vi "WRITE CAN DATA DBL.vi"(7 "Enum":T1=enum."GET", 8 "error in (no error)":errorcluster, 11 "CAN DATA IN":dbl[](array[numeric])) -> (0 "error out":errorcluster, 3 "CAN DATA OUT":dbl[](array[numeric]))   [LabVIEW 2018]
uses:
  Controls/READ CAN DATA.ctl
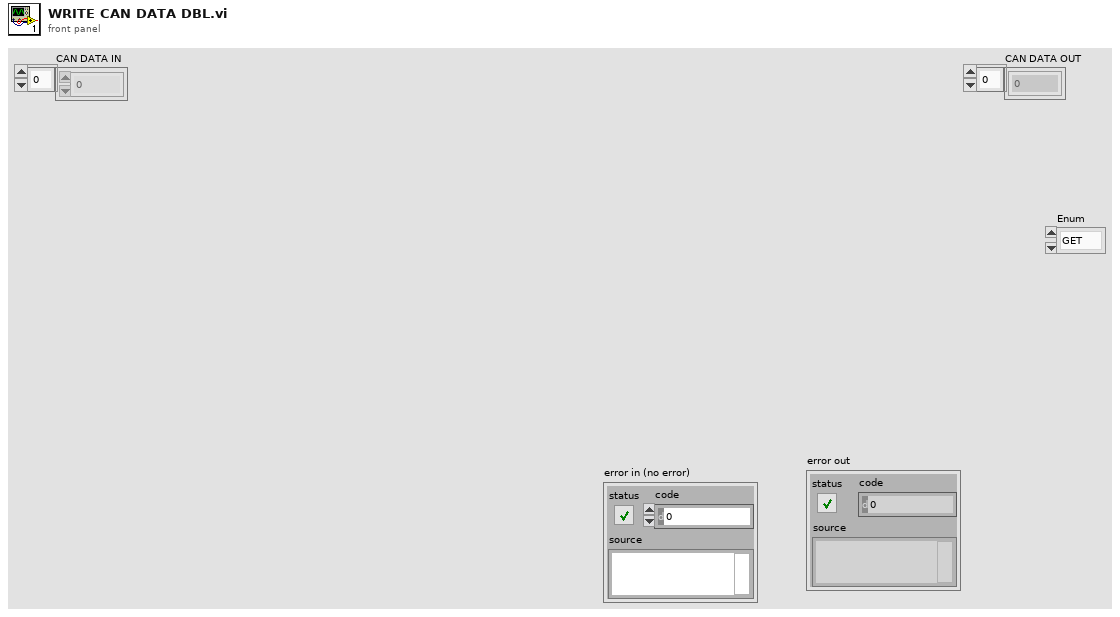
[diagram p1: front panel]
types:
  T1 = typedef "READ CAN DATA.ctl" = enum16{"SET", "GET"}
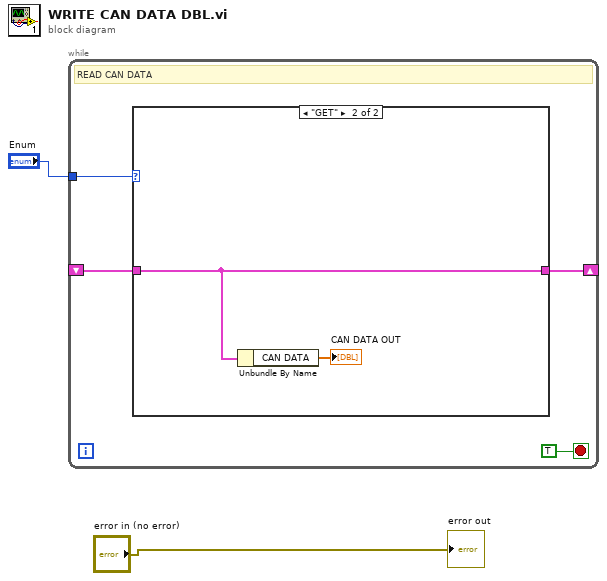
[diagram p0: block diagram]
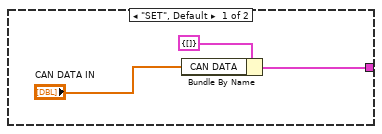
[diagram p2: hidden frame]
diagram:
  n1 = while {
    tunnel: "Enum" -> [w5]
    shift-right: [w4] -> _
    shift-left: _ -> [w3]
    stop <- TRUE stop-if-true
    # "READ CAN DATA"
    n2 = case shown="\"GET\"" w5 {
      tunnel: [w8 w11] -> w4
      tunnel: w3 -> [_ w11]
      frame "SET", Default {
        n3 = Bundle By Name(cluster=cluster{"CAN DATA":dbl[]} {"CAN DATA"=[]}, "CAN DATA"="CAN DATA IN") -> (w8:cluster{"CAN DATA":dbl[]})
      }
      frame "GET" {
        n4 = Unbundle By Name(w11) -> ("CAN DATA"=→"CAN DATA OUT":dbl[])
      }
    }
  }
  "error out" <- "error in (no error)"
